vi "DereferencingPointerToArrayOfSimpleStructUsingMoveBlock.vi"(8 "error in (no error)":errorcluster, 10 "Length":i32, 11 "Address (Pointer)":i64) -> (0 "error out":errorcluster, 3 "Destination":T1[](array[typedef]))   [LabVIEW 2009, in "LabVIEWWrapper_PassingDataSampleDLL.lvlib"]
uses:
  LabVIEWWrapper_PassingDataSampleDLL.lvlib
  CustomControlsForStructs/SimpleStruct Circle.ctl
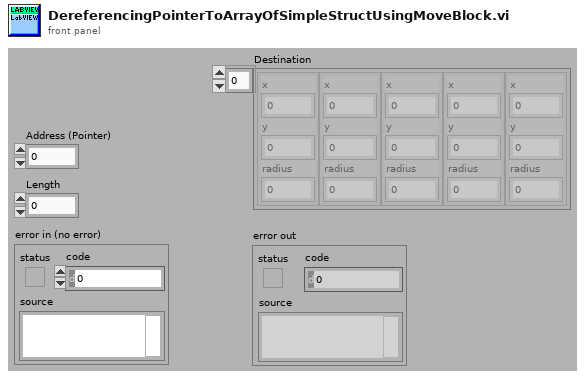
[diagram p1: front panel]
types:
  T1 = typedef "LabVIEWWrapper_PassingDataSampleDLL.lvlib/SimpleStruct Circle.ctl" = cluster{"x":sgl, "y":sgl, "radius":sgl}
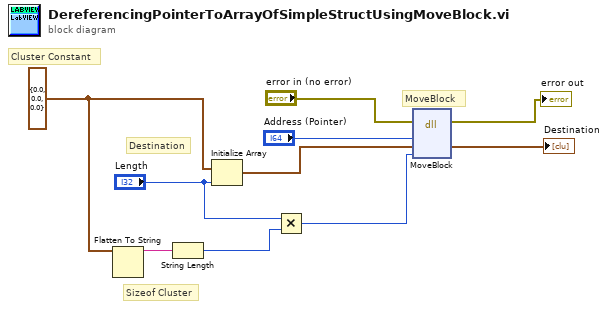
[diagram p0: block diagram]
diagram:
  w3 = cluster{"x":sgl, "y":sgl, "radius":sgl} {"x"=0.0, "y"=0.0, "radius"=0.0} ("Circle")
  # "Cluster Constant"
  # "Sizeof Cluster"
  # "Destination"
  # "MoveBlock"
  n1 = Flatten To String(anything=w3) -> (data string=w2:string)  [unwired: 3 in, 2 out]
  n2 = String Length(string=w2) -> (length=w1:i32)
  n3 = Initialize Array(w3, "Length") -> (w7:cluster{"x":sgl, "y":sgl, "radius":sgl}[])
  n4 = Multiply(x="Length", y=w1) -> (x*y=w4:i32)
  n5 = dll-call lib="LabVIEW" fn="MoveBlock"(error in="error in (no error)", "Address (Pointer)"="Address (Pointer)", "Destination"=w7, "Size"=w4) -> (error out=→"error out":errorcluster, "Destination"=→"Destination":cluster{"x":sgl, "y":sgl, "radius":sgl}[])  [unwired: 5 in, 1 out]
